vi "Search for Barrels.vi"(8 "error in (no error)":errorcluster) -> (0 "error out":errorcluster, 2 "Observed LM Array":T1(array[cluster]), 4 "RAW SICK":cluster{dbl[], dbl[]})   [LabVIEW 2009]
uses:
  <vilib>/Analysis/Matrix/Datatypes/RealMatrix.ctl
  TypeDefs/Sensor TypeDefs/SICK Array.ctl
  <vilib>/Analysis/baseanly.llb/Real A x B.vi
  <vilib>/Analysis/Matrix/NI_Matrix.lvlib
  <vilib>/Analysis/NI_AALBase.lvlib
panel:
  out "Number of Barrels":i32=2
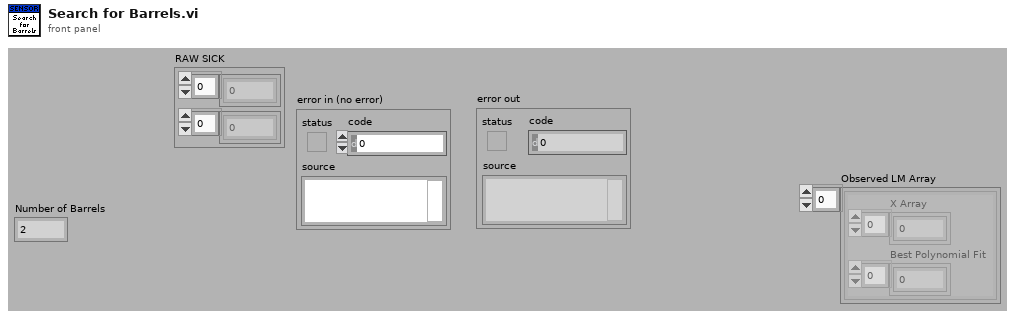
[diagram p1: front panel]
types:
  T1 = cluster{"X Array":dbl[], "Best Polynomial Fit":dbl[]}[]
  T2 = typedef "NI_Matrix.lvlib/RealMatrix.ctl" = dbl[][]
  T3 = typedef "SICK Array.ctl" = u16[]
  T4 = cluster{"Rotated Array":cluster{"X":dbl, "Y":dbl}[]}[]
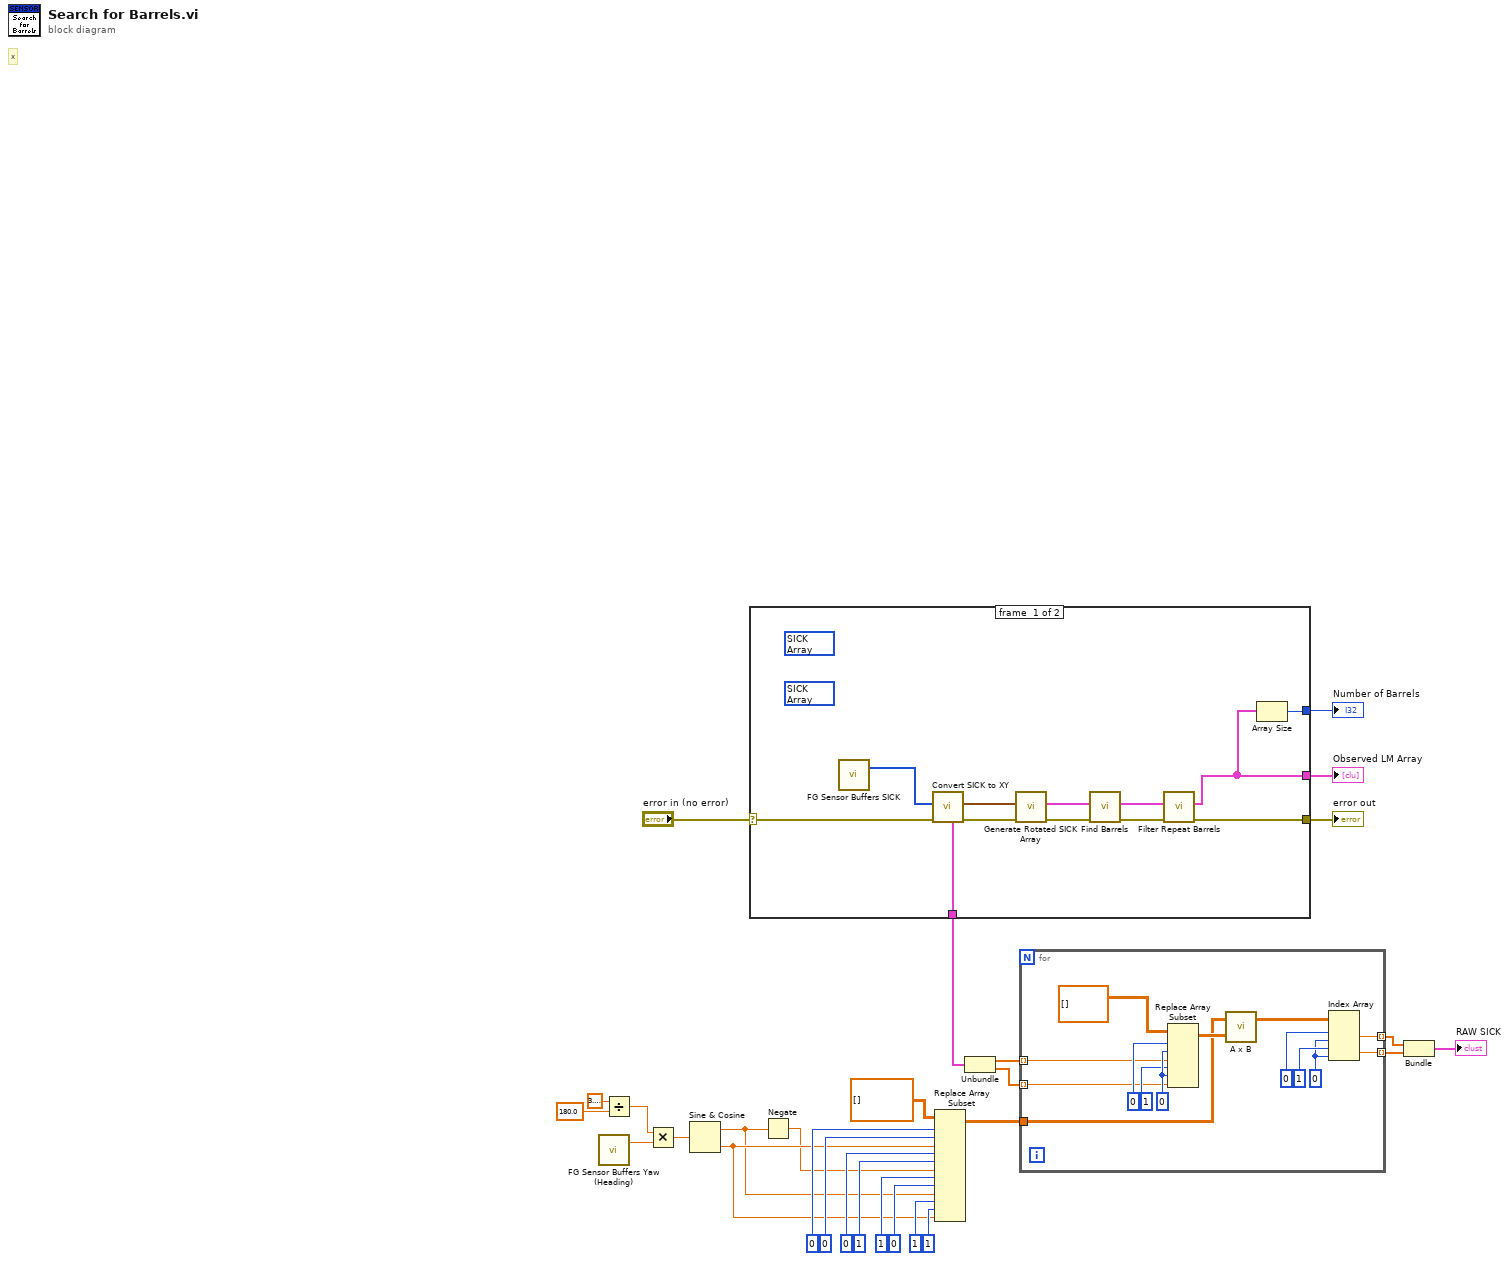
[diagram p0: block diagram]
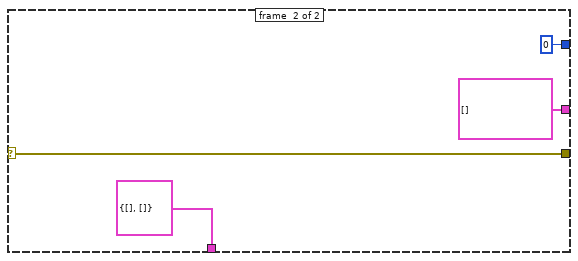
[diagram p2: hidden frame]
diagram:
  # "x"
  n1 = call "FG Sensor Buffers Yaw (Heading).vi"() -> ("Yaw Buffer Out"=w21:dbl)  [unwired: 3 in]
  n2 = Divide(x=3.141592653589793, y=180.0) -> (x/y=w22:dbl)
  n3 = Multiply(x=w22, y=w21) -> (x*y=w8:dbl)
  n4 = Sine & Cosine(0:w8) -> (1:w11:dbl, 2:w12:dbl)
  n5 = case shown="No Error" "error in (no error)" {
    selector: "error in (no error)" -> [w30 w44]
    tunnel: [w40 0] -> w28
    tunnel: [w39 T1 [] ("Observed LM Array")] -> w27
    tunnel: [w38 w44] -> w26
    tunnel: [w29 cluster{dbl[], dbl[]} {[], []} ("RAW SICK")] -> w7
    frame #0 {
      (unwired) T3 [544, 544, 544, 544, 544, 545, 549, 553, 563, 614, 617, 630, 379, 341, 311, 310, 313, 314, 316, 317, 318, 319, 576, 579, 583, 587, 592, 596, 601, 606, 611, 617, 624, 628, 635, 642, 649, 656, 664, 673, 682, 691, 700, 711, 722, 733, 746, 757, 771, 785, 799, 815, 830, 847, 865, 2237, 2846, 2121, 2967, 2153, 1952, 1952, 2152, 2134, 2194, 2190, 2177, 2232, 8191, 4486, 4643, 4673, 4649, 8191, 8191, 3590, 3878, 3790, 3809, 8191, 8191, 8191, 333, 324, 319, 317, 316, 317, 320, 325, 335, 8191, 327, 321, 316, 316, 316, 317, 319, 325, 8191, 339, 331, 328, 326, 324, 326, 329, 335, 8191, 8191, 8191, 8191, 8191, 8191, 3824, 3865, 3431, 3491, 3500, 3757, 3184, 3129, 3145, 3733, 3171, 3082, 3065, 3098, 2971, 3069, 3764, 3450, 3471, 3558, 8191, 3138, 3086, 3004, 3203, 2857, 2848, 2993, 2903, 2883, 8191, 8191, 8191, 8191, 8191, 8191, 8183, 8191, 8191, 8191, 8191, 8191, 8191, 242, 239, 238, 238, 236, 234, 233, 231, 228, 227, 234, 251, 270, 291, 267, 8191, 8191, 8191, 8191, 8191, 8191, 8191, 8191] ("SICK Data 2")
      (unwired) T3 [154, 155, 155, 103, 96, 95, 95, 95, 95, 95, 95, 95, 96, 97, 99, 102, 110, 130, 130, 132, 134, 135, 136, 138, 140, 142, 142, 144, 146, 148, 150, 152, 153, 157, 158, 162, 164, 167, 170, 173, 177, 189, 195, 491, 486, 481, 476, 471, 468, 449, 446, 442, 440, 436, 434, 431, 428, 425, 423, 421, 418, 416, 292, 283, 280, 279, 278, 278, 280, 282, 287, 305, 306, 283, 279, 276, 274, 274, 275, 277, 279, 286, 405, 406, 407, 408, 410, 412, 414, 416, 417, 419, 421, 423, 425, 428, 431, 434, 437, 440, 443, 179, 160, 152, 145, 137, 131, 125, 121, 116, 111, 107, 104, 101, 97, 94, 91, 89, 86, 85, 320, 319, 89, 8191, 135, 135, 140, 123, 119, 117, 117, 119, 120, 125, 123, 127, 128, 126, 125, 125, 125, 127, 126, 126, 128, 128, 133, 226, 225, 224, 218, 228, 263, 393, 395, 395, 394, 384, 561, 550, 559, 567, 576, 322, 316, 316, 316, 319, 320, 323, 336, 341, 424, 578, 572, 582, 583, 265, 261, 525, 531] ("reversed array")
      n6 = call "FG Sensor Buffers SICK.vi"() -> ("SICK Buffer out"=w37:T3)  [unwired: 3 in]
      n7 = call "Convert SICK to XY.vi"("error in (no error)"=w30, "SICK Buffer"=w37) -> ("error out"=w36:errorcluster, "Close SICK"=w35:cluster{"x":dbl, "y":dbl}[], "RAW SICK"=w29:cluster{dbl[], dbl[]})  [unwired: 7 in]
      n8 = call "Generate Rotated SICK Array.vi"("error in (no error)"=w36, "Close SICK"=w35) -> ("error out"=w34:errorcluster, "Rotated SICK Array"=w33:T4)  [unwired: 8 in]
      n9 = call "Find Barrels.vi"("error in (no error)"=w34, "Rotated SICK Array"=w33) -> ("error out"=w32:errorcluster, "Barrels"=w31:T1)  [unwired: 8 in]
      n10 = call "Filter Repeat Barrels.vi"("error in (no error)"=w32, "Barrel Array"=w31) -> ("error out"=w38:errorcluster, "Observed LM Array"=w39:T1)  [unwired: 8 in]
      n11 = Array Size(array=w39) -> (size(s)=w40:i32)
    }
    frame #1 {
    }
  }
  "error out" <- w26
  "Observed LM Array" <- w27
  "Number of Barrels" <- w28
  n12 = Negate(x=w11) -> (-x=w10:dbl)
  n13 = Replace Array Subset(array=T2 [] ("matrix"), new element #1=w12, index (row) #1=0 ("disabled index (row)"), index (col) #1=0 ("disabled index (row)"), new element #2=w10, index (row) #2=0 ("disabled index (row)"), index (col) #2=1 ("disabled index (row)"), new element #3=w11, index (row) #3=1 ("disabled index (row)"), index (col) #3=0 ("disabled index (row)"), new element #4=w12, index (row) #4=1 ("disabled index (row)"), index (col) #4=1 ("disabled index (row)")) -> (w6:T2)
  n14 = Unbundle(w7) -> (w5:dbl[], w4:dbl[])
  n15 = for {
    tunnel: w6 -> [w49]
    tunnel: w5 -> [w48] mode=indexing
    tunnel: w4 -> [w47] mode=indexing
    tunnel: [w46] -> w2 mode=indexing
    tunnel: [w45] -> w3 mode=indexing
    w51 = 0 ("index (col)")
    w57 = 0 ("index (col)")
    n16 = Replace Array Subset(array=T2 [] ("matrix"), new element #1=w48, index (row) #1=0 ("index (col)"), index (col) #1=w57, new element #2=w47, index (row) #2=1 ("index (col)"), index (col) #2=w57) -> (w54:T2)
    n17 = call-poly <vilib>:"A x B.vi"("B"=w54, "A"=w49) -> ("A x B"=w50:T2)  [unwired: 1 out]
    n18 = Index Array(array=w50, index (row) #1=0 ("index (col)"), index (col) #1=w51, index (row) #2=1 ("index (col)"), index (col) #2=w51) -> (element #1=w46:dbl, element #2=w45:dbl)
  }
  n19 = Bundle(w2, w3) -> (→"RAW SICK":cluster{dbl[], dbl[]})  [unwired: 1 in]
